vi "Disabled.vi"(7 "Robot Mode":T2, 10 "Match Info":T1={"Autonomous Elapsed Seconds"=0.0, "TeleOp Elapsed Seconds"=0.0, "Disabled Elapsed Seconds"=0.0, "Visited Autonomous"=FALSE, "Visited TeleOp"=FALSE, "Visited Disabled"=FALSE, "Autonomous Settings"={"Autonomous Style"=enum."Independent", "VI Refnum"=refnum}}, 11 "Call Context":T3) -> ()   [LabVIEW 2019]
doc: "This VI is called each time a disabled packet is received from the DS. It can be used to prepare for the next robot mode, to calibrate sensors, etc."
uses:
  <vilib>/Rock Robotics/WPI/DriverStation/WPI_DriverStationDerivedRobotMode.ctl
  <vilib>/Rock Robotics/WPI/DriverStation/WPI_DriverStationRobotMode2.ctl
  <vilib>/Rock Robotics/WPI/DriverStation/WPI_DriverStationMatch Info.ctl
  <vilib>/Rock Robotics/WPI/Joystick/WPI_JoystickDeviceEnum.ctl
  <vilib>/Rock Robotics/WPI/Utilities/WPI_GetSetVariantRefNum.vi
  <vilib>/Rock Robotics/WPI/Joystick/WPI_JoystickXBox Types.ctl
  Support Code/Indicator LED Indexes.ctl
  Support Code/Indicator LED - Red.ctl
  Support Code/Indicator LED - Green.ctl
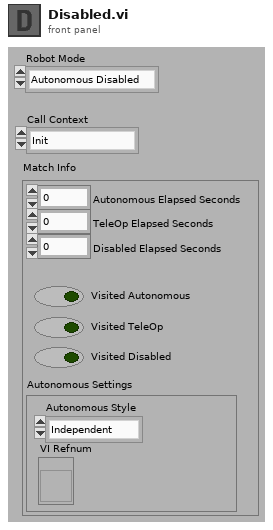
[diagram p1: front panel]
types:
  T1 = typedef "WPI_DriverStationMatch Info.ctl" = cluster{"Autonomous Elapsed Seconds":dbl, "TeleOp Elapsed Seconds":dbl, "Disabled Elapsed Seconds":dbl, "Visited Autonomous":bool, "Visited TeleOp":bool, "Visited Disabled":bool, "Autonomous Settings":cluster{"Autonomous Style":enum16{"Iterative", "Independent"}, "VI Refnum":refnum<vi>}}
  T2 = typedef "WPI_DriverStationRobotMode2.ctl" = enum16{"Autonomous Disabled", "Autonomous Enabled", "Teleop Disabled", "Teleop Enabled", "Disconnected", "Finish", "Test Disabled", "Test Enabled", "Emergency Stopped"}
  T3 = typedef "WPI_DriverStationDerivedRobotMode.ctl" = enum16{"Init", "Execute", "Stop"}
  T4 = typedef "WPI_JoystickXBox Types.ctl" = enum16{"Not XBox", "XBox Unknown", "XBox Gamepad", "XBox Wheel", "XBox Arcade Stick", "XBox Flight Stick", "XBox Dance Pad", "XBox Guitar", "XBox Drum Kit", "XBox Arcade Pad"}
  T5 = typedef "WPI_JoystickDeviceEnum.ctl" = enum16{"USB 0", "USB 1", "USB 2", "USB 3", "USB 4", "USB 5"}
  T6 = typedef "WPI_JoystickDevRef.ctl" = cluster{"Device":T5}
  T7 = typedef "WPI_Joystick Info.ctl" = cluster{"Device Name":string, "HID Type":T8, "XBox Type":T4, "Axes Count":i32, "Axes Types":T9[], "Button Count":i32, "POV Count":i32}
  T8 = typedef "WPI_JoystickHID Types.ctl" = enum16{"Not HID", "HID Joystick", "HID Gamepad", "HID Driving Wheel", "HID Flightstick", "HID First Person"}
  T9 = typedef "WPI_JoystickAxis Types.ctl" = enum16{"X Axis", "Y Axis", "Z Axis", "RxAxis", "RyAxis", "RzAxis", "Slider", "POV", "None", "L X Axis", "L Y Axis", "L Trigger", "R Trigger", "R X Axis", "R Y Axis"}
  T10 = typedef "Indicator LED - Red.ctl" = u32
  T11 = typedef "Indicator LED Indexes.ctl" = enum16{"Code Started", "DS Connected", "Limelight", "Turret Calibrated", "Gyro Calibrated", "USB0 Connected", "USB1 Connected"}
  T12 = typedef "Indicator LED - Green.ctl" = u32
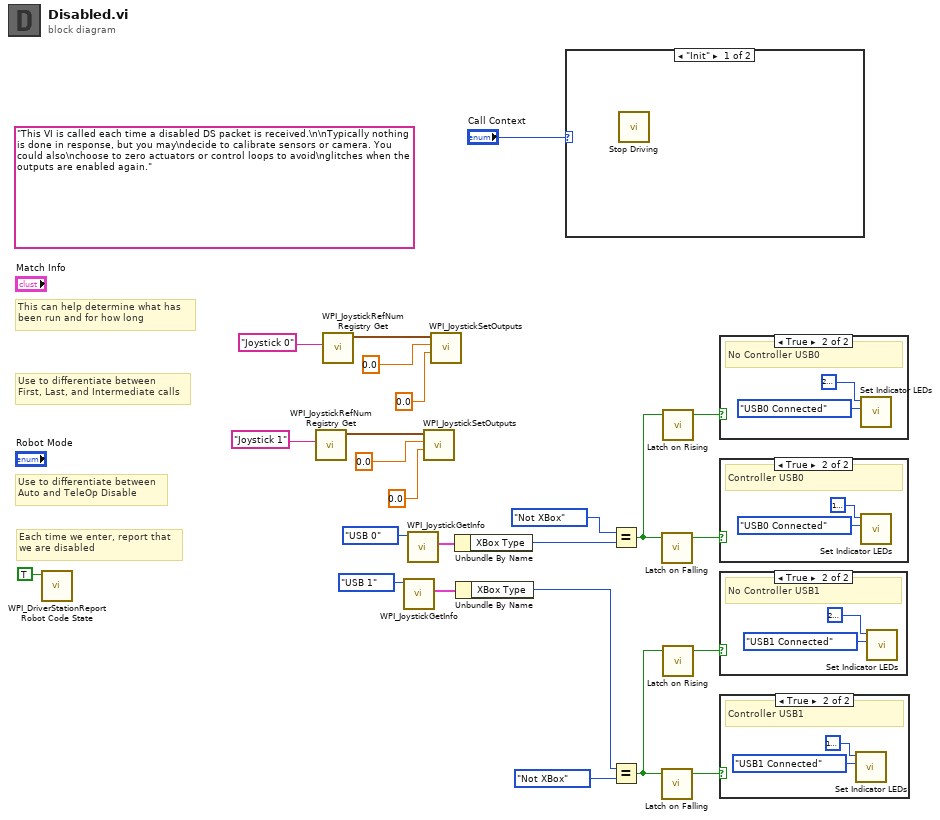
[diagram p0: block diagram]
diagram:
  (unwired) "This VI is called each time a disabled DS packet is received.\n\nTypically nothing is done in response, but you may\ndecide to calibrate sensors or camera. You could also\nchoose to zero actuators or control loops to avoid\nglitches when the outputs are enabled again."
  # "Each time we enter, report that\nwe are disabled"
  # "Use to differentiate between\nFirst, Last, and Intermediate calls"
  # "This can help determine what has\nbeen run and for how long"
  # "Use to differentiate between\nAuto and TeleOp Disable"
  n1 = call <vilib>:"WPI_DriverStationReport Robot Code State.vi"("Disabled"=TRUE ("Autonomous")) -> ()  [unwired: 10 in, 1 out]
  n2 = call <vilib>:"WPI_JoystickRefNum Registry Get.vi"("refnum name"="Joystick 1") -> ("JoystickDevRef"=w18:T6)  [unwired: 1 in, 9 out]
  n3 = call <vilib>:"WPI_JoystickRefNum Registry Get.vi"("refnum name"="Joystick 0") -> ("JoystickDevRef"=w19:T6)  [unwired: 1 in, 9 out]
  n4 = call <vilib>:"WPI_JoystickGetInfo.vi"("JoystickDevice"=WPI_JoystickDeviceEnum."USB 1") -> ("Joystick Info"=w11:T7)  [unwired: 9 in, 1 out]
  n5 = call <vilib>:"WPI_JoystickGetInfo.vi"("JoystickDevice"=WPI_JoystickDeviceEnum."USB 0") -> ("Joystick Info"=w12:T7)  [unwired: 9 in, 1 out]
  n6 = call <vilib>:"WPI_JoystickSetOutputs.vi"("Right Rumble"=sgl 0.0, "Left Rumble"=sgl 0.0, "JoystickDevRef"=w18) -> ()  [unwired: 7 in, 2 out]
  n7 = call <vilib>:"WPI_JoystickSetOutputs.vi"("Right Rumble"=sgl 0.0, "Left Rumble"=sgl 0.0, "JoystickDevRef"=w19) -> ()  [unwired: 7 in, 2 out]
  n8 = Unbundle By Name(w12) -> ("XBox Type"=w10:T4)
  n9 = Unbundle By Name(w11) -> ("XBox Type"=w1:T4)
  n10 = case shown="\"Init\"" "Call Context" {
    frame "Init" {
      n11 = call "Stop Driving.vi"() -> ()  [unwired: 11 in, 1 out]
    }
    frame "Execute", Default {
    }
  }
  n12 = Equal?(x=WPI_JoystickXBox_Types."Not XBox", y=w10) -> (x = y?=w8:bool)
  n13 = Equal?(x=w1, y=WPI_JoystickXBox_Types."Not XBox" ("x")) -> (x = y?=w3:bool)
  n14 = call <vilib>:"Latch on Falling.vi"("Boolean in"=w8) -> ("Boolean out"=w6:bool)  [unwired: 4 in]
  n15 = call <vilib>:"Latch on Falling.vi"("Boolean in"=w3) -> ("Boolean out"=w5:bool)  [unwired: 4 in]
  n16 = call <vilib>:"Latch on Rising.vi"("Boolean in"=w8) -> ("Boolean out"=w7:bool)  [unwired: 4 in]
  n17 = call <vilib>:"Latch on Rising.vi"("Boolean in"=w3) -> ("Boolean out"=w4:bool)  [unwired: 4 in]
  n18 = case shown="True" w7 {
    frame False {
    }
    frame True {
      # "No Controller USB0"
      n19 = call "Set Indicator LEDs.vi"("LED Index"=Indicator_LED_Indexes."USB0 Connected", "Color"=T10 2490368) -> ()  [unwired: 9 in, 1 out]
    }
  }
  n20 = case shown="True" w6 {
    frame False {
    }
    frame True {
      # "Controller USB0"
      n21 = call "Set Indicator LEDs.vi"("LED Index"=Indicator_LED_Indexes."USB0 Connected", "Color"=T12 1851904) -> ()  [unwired: 9 in, 1 out]
    }
  }
  n22 = case shown="True" w4 {
    frame False {
    }
    frame True {
      # "No Controller USB1"
      n23 = call "Set Indicator LEDs.vi"("LED Index"=Indicator_LED_Indexes."USB1 Connected", "Color"=T10 2490368) -> ()  [unwired: 9 in, 1 out]
    }
  }
  n24 = case shown="True" w5 {
    frame False {
    }
    frame True {
      # "Controller USB1"
      n25 = call "Set Indicator LEDs.vi"("LED Index"=Indicator_LED_Indexes."USB1 Connected", "Color"=T12 1851904) -> ()  [unwired: 9 in, 1 out]
    }
  }
